vi "Close.vi"(8 "error in (no error)":errorcluster, 10 "Return Code":i32) -> (0 "error out":errorcluster)   [LabVIEW 2017, in "MGI-Console.lvlib" / "Console.lvclass"]
doc: "Closes the console and application. Non-zero return codes typically mean there was an error.\n----\nCopyright: MGI 2018\nAuthor: Derek Trepanier"
uses:
  Console.lvclass
  msvcrt.dll
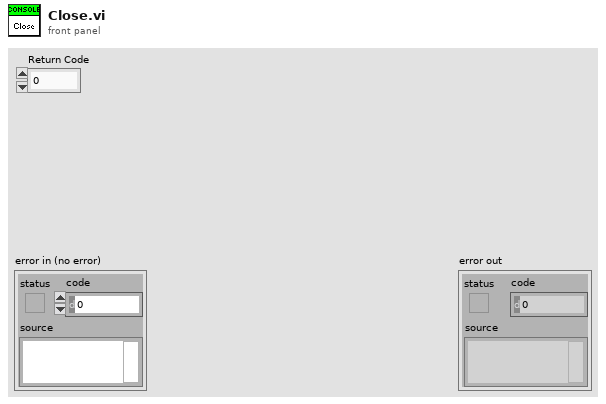
[diagram p1: front panel]
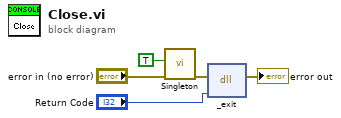
[diagram p0: block diagram]
diagram:
  n1 = call "Singleton.vi"("error in (no error)"="error in (no error)", "Close?"=TRUE) -> ("error out"=w3:errorcluster)  [unwired: 9 in]
  n2 = dll-call lib="msvcrt.dll" fn="_exit"(error in=w3, "code"="Return Code") -> (error out=→"error out":errorcluster)  [unwired: 4 in, 1 out]
